vi "2 line get round smallest r center.vi"(1 "D":cluster{dbl, dbl}, 2 "C":cluster{dbl, dbl}, 3 "B":cluster{dbl, dbl}, 4 "A":cluster{dbl, dbl}) -> (0 "small R center":cluster{dbl, dbl})   [LabVIEW 2019]
panel:
  out "XY Graph":cluster{cluster{dbl, dbl}[]}[](graph)
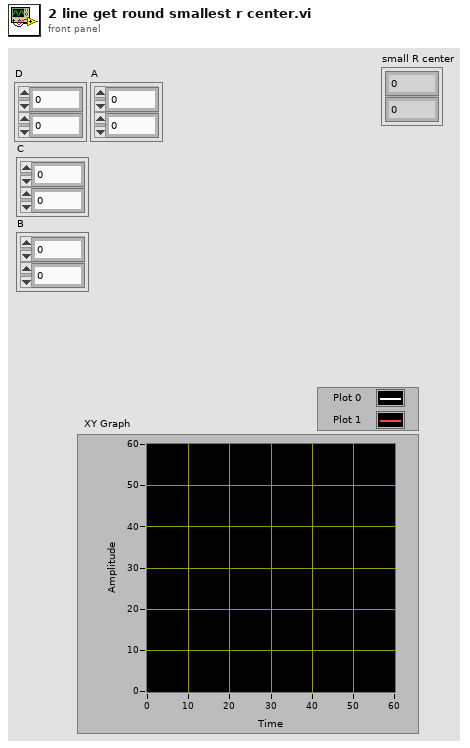
[diagram p1: front panel]
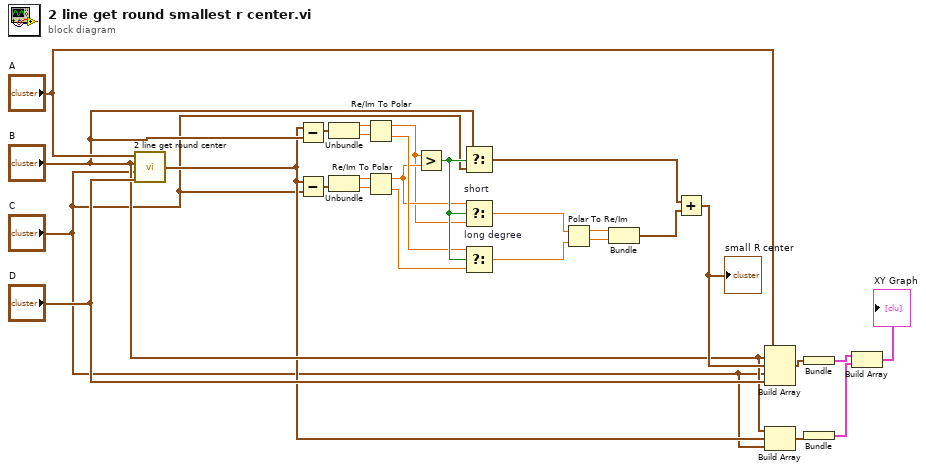
[diagram p0: block diagram]
diagram:
  n1 = call "2 line get round center.vi"("D"="D", "C"="C", "B"="B", "A"="A") -> ("round center"=w4:cluster{dbl, dbl})
  n2 = Subtract(x=w4, y="B") -> (x-y=w22:cluster{dbl, dbl})
  n3 = Subtract(x=w4, y="C") -> (x-y=w24:cluster{dbl, dbl})
  n4 = Unbundle(w22) -> (w28:dbl, w27:dbl)
  n5 = Unbundle(w24) -> (w25:dbl, w26:dbl)
  n6 = Re/Im To Polar(2:w27, 3:w28) -> (0:w13:dbl, 1:w10:dbl)
  n7 = Re/Im To Polar(2:w26, 3:w25) -> (0:w12:dbl, 1:w11:dbl)
  n8 = Greater?(x=w10, y=w11) -> (0:w23:bool)
  n9 = Select(t="B", s=w23, f="C") -> (s? t:f=w18:cluster{dbl, dbl})
  n10 = Select "short"(t=w11, s=w23, f=w10) -> (s? t:f=w9:dbl)
  n11 = Select "long degree"(t=w13, s=w23, f=w12) -> (s? t:f=w8:dbl)
  n12 = Polar To Re/Im(2:w8, 3:w9) -> (0:w21:dbl, 1:w20:dbl)
  n13 = Bundle(w20, w21) -> (w19:cluster{dbl, dbl})  [unwired: 1 in]
  n14 = Add(x=w18, y=w19) -> (x+y=w17:cluster{dbl, dbl})
  "small R center" <- w17
  n15 = Build Array("A", "B", w17, "C", "D") -> (w16:cluster{dbl, dbl}[])
  n16 = Build Array("B", w4, "C") -> (w2:cluster{dbl, dbl}[])
  n17 = Bundle(w16) -> (w15:cluster{cluster{dbl, dbl}[]})  [unwired: 1 in]
  n18 = Bundle(w2) -> (w1:cluster{cluster{dbl, dbl}[]})  [unwired: 1 in]
  n19 = Build Array(w15, w1) -> (→"XY Graph":cluster{cluster{dbl, dbl}[]}[])
